vi "Read StateRef.vi"(8 "error in (no error)":errorcluster, 11 "XBoxController in":refnum<class "XBoxController.lvclass">) -> (0 "error out":errorcluster, 2 "StateRef":refnum<vi>, 3 "XBoxController out":refnum<class "XBoxController.lvclass">)   [LabVIEW 2013]
uses:
  XBoxController.lvclass
  XBoxJoystick.ctl
  State.ctl
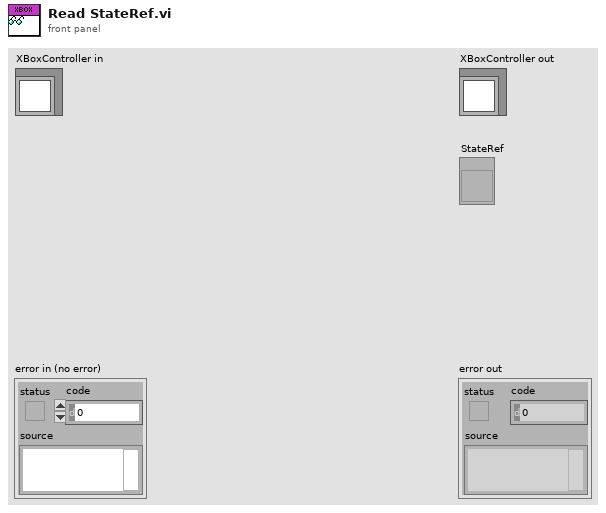
[diagram p1: front panel]
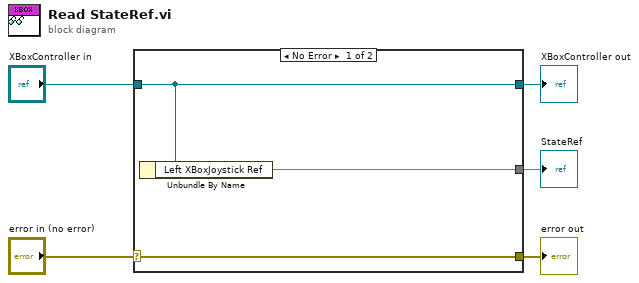
[diagram p0: block diagram]
diagram:
  n1 = case shown="No Error" "error in (no error)" {
    selector: "error in (no error)" -> [w8 w9]
    tunnel: [w8 w9] -> w4
    tunnel: [w7 w10] -> w2
    tunnel: "XBoxController in" -> [w7 w10]
    tunnel: [w6 _] -> w1
    frame No Error {
      n2 = Unbundle By Name(w7) -> ("Left XBoxJoystick Ref"=w6)
    }
    frame Error {
    }
  }
  "error out" <- w4
  "XBoxController out" <- w2
  "StateRef" <- w1
